vi "PCO_Convert.vi"() -> (1 "Raw_Length":u16, 4 "Length":u16, 6 "PCO_ConvertRaw_x64":T2, 7 "PCO_ConvertRaw_win32":T1, 8 "PCO_Convert":T3)   [LabVIEW 2019, in "Convert.lvlib"]
doc: "Use this template to build a VI to use as a subVI."
uses:
  Convert.lvlib
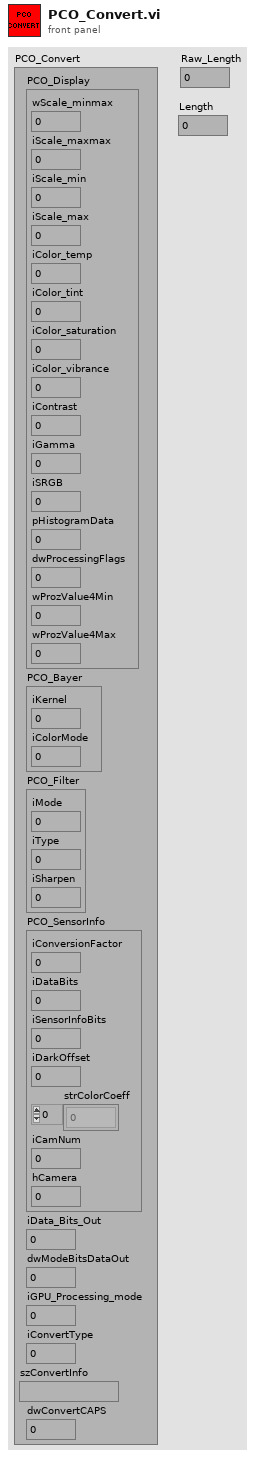
[diagram p1: front panel]
types:
  T1 = cluster{"wSize":u16, "wDummy":cluster{u16, u16, u16}, "PCO_DisplayRaw_win32":cluster{"wSize":u16, "wScale_minmax":u16, "iScale_maxmax":i32, "iScale_min":i32, "iScale_max":i32, "iColor_temp":i32, "iColor_tint":i32, "iColor_saturation":i32, "iColor_vibrance":i32, "iContrast":i32, "iGamma":i32, "iSRGB":i32, "pHistogramData":u32, "dwDialogOpenFlags":u32, "dwProcessingFlags":u32, "wProzValue4Min":u16, "wProzValue4Max":u16, "dwzzDummy1":cluster{u32, u32, u32, u32, u32, u32, u32, u32, u32, u32, u32, u32, u32, u32, u32, u32, u32, u32, u32, u32, u32, u32, u32, u32, u32, u32, u32, u32, u32, u32, u32, u32, u32, u32, u32, u32, u32, u32, u32, u32, u32, u32, u32, u32, u32, u32, u32, u32, u32}}, "PCO_Bayer_Raw":cluster{"wSize":u16, "wDummy":u16, "iKernel":i32, "iColorMode":i32, "dwzzDummy1":cluster{u32, u32, u32, u32, u32, u32, u32, u32, u32, u32, u32, u32, u32, u32, u32, u32, u32, u32, u32, u32, u32, u32, u32, u32, u32, u32, u32, u32, u32, u32, u32, u32, u32, u32, u32, u32, u32, u32, u32, u32, u32, u32, u32, u32, u32, u32, u32, u32, u32, u32, u32, u32, u32, u32, u32, u32, u32, u32, u32, u32, u32}}, "PCO_Filter_Raw":cluster{"wSize":u16, "wDummy":u16, "iMode":i32, "iType":i32, "iSharpen":i32, "dwzzDummy1":cluster{u32, u32, u32, u32, u32, u32, u32, u32, u32, u32, u32, u32, u32, u32, u32, u32, u32, u32, u32, u32, u32, u32, u32, u32, u32, u32, u32, u32, u32, u32, u32, u32, u32, u32, u32, u32, u32, u32, u32, u32, u32, u32, u32, u32, u32, u32, u32, u32, u32, u32, u32, u32, u32, u32, u32, u32, u32, u32, u32, u32}}, "PCO_SensorInfo_Raw_win32":cluster{"wSize":u16, "wDummy":u16, "iConversionFactor":i32, "iDataBits":i32, "iSensorInfoBits":i32, "iDarkOffset":i32, "dwzzDummy0":u32, "strColorCoeff":cluster{dbl, dbl, dbl, dbl, dbl, dbl, dbl, dbl, dbl}, "iCamNum":i32, "hCamera":u32, "dwzzDummy1":cluster{u32, u32, u32, u32, u32, u32, u32, u32, u32, u32, u32, u32, u32, u32, u32, u32, u32, u32, u32, u32, u32, u32, u32, u32, u32, u32, u32, u32, u32, u32, u32, u32, u32, u32, u32, u32, u32, u32}}, "iData_Bits_Out":i32, "dwModeBitsDataOut":u32, "iGPU_Processing_mode":i32, "iConvertType":i32, "szConvertInfo":cluster{u8, u8, u8, u8, u8, u8, u8, u8, u8, u8, u8, u8, u8, u8, u8, u8, u8, u8, u8, u8, u8, u8, u8, u8, u8, u8, u8, u8, u8, u8, u8, u8, u8, u8, u8, u8, u8, u8, u8, u8, u8, u8, u8, u8, u8, u8, u8, u8, u8, u8, u8, u8, u8, u8, u8, u8, u8, u8, u8, u8}, "dwConvertCAPS":u32, "dwzzDummy1":cluster{u32, u32, u32, u32, u32, u32, u32, u32, u32, u32, u32, u32, u32, u32, u32, u32, u32, u32, u32, u32, u32, u32, u32, u32, u32, u32, u32, u32, u32, u32, u32, u32, u32, u32, u32, u32, u32, u32, u32, u32, u32, u32}}
  T2 = cluster{"wSize":u16, "wDummy":cluster{u16, u16, u16}, "PCO_DisplayRaw_x64":cluster{"wSize":u16, "wScale_minmax":u16, "iScale_maxmax":i32, "iScale_min":i32, "iScale_max":i32, "iColor_temp":i32, "iColor_tint":i32, "iColor_saturation":i32, "iColor_vibrance":i32, "iContrast":i32, "iGamma":i32, "iSRGB":i32, "pHistogramData":u64, "dwDialogOpenFlags":u32, "dwProcessingFlags":u32, "wProzValue4Min":u16, "wProzValue4Max":u16, "dwzzDummy1":cluster{u32, u32, u32, u32, u32, u32, u32, u32, u32, u32, u32, u32, u32, u32, u32, u32, u32, u32, u32, u32, u32, u32, u32, u32, u32, u32, u32, u32, u32, u32, u32, u32, u32, u32, u32, u32, u32, u32, u32, u32, u32, u32, u32, u32, u32, u32, u32, u32, u32, u32}}, "PCO_Bayer_Raw":cluster{"wSize":u16, "wDummy":u16, "iKernel":i32, "iColorMode":i32, "dwzzDummy1":cluster{u32, u32, u32, u32, u32, u32, u32, u32, u32, u32, u32, u32, u32, u32, u32, u32, u32, u32, u32, u32, u32, u32, u32, u32, u32, u32, u32, u32, u32, u32, u32, u32, u32, u32, u32, u32, u32, u32, u32, u32, u32, u32, u32, u32, u32, u32, u32, u32, u32, u32, u32, u32, u32, u32, u32, u32, u32, u32, u32, u32, u32}}, "PCO_Filter_Raw":cluster{"wSize":u16, "wDummy":u16, "iMode":i32, "iType":i32, "iSharpen":i32, "dwzzDummy1":cluster{u32, u32, u32, u32, u32, u32, u32, u32, u32, u32, u32, u32, u32, u32, u32, u32, u32, u32, u32, u32, u32, u32, u32, u32, u32, u32, u32, u32, u32, u32, u32, u32, u32, u32, u32, u32, u32, u32, u32, u32, u32, u32, u32, u32, u32, u32, u32, u32, u32, u32, u32, u32, u32, u32, u32, u32, u32, u32, u32, u32}}, "PCO_SensorInfo_Raw_x64":cluster{"wSize":u16, "wDummy":u16, "iConversionFactor":i32, "iDataBits":i32, "iSensorInfoBits":i32, "iDarkOffset":i32, "dwzzDummy0":u32, "strColorCoeff":cluster{dbl, dbl, dbl, dbl, dbl, dbl, dbl, dbl, dbl}, "iCamNum":i32, "hCamera":u64, "dwzzDummy1":cluster{u32, u32, u32, u32, u32, u32, u32, u32, u32, u32, u32, u32, u32, u32, u32, u32, u32, u32, u32, u32, u32, u32, u32, u32, u32, u32, u32, u32, u32, u32, u32, u32, u32, u32, u32, u32, u32, u32, u32}}, "iData_Bits_Out":i32, "dwModeBitsDataOut":u32, "iGPU_Processing_mode":i32, "iConvertType":i32, "szConvertInfo":cluster{u8, u8, u8, u8, u8, u8, u8, u8, u8, u8, u8, u8, u8, u8, u8, u8, u8, u8, u8, u8, u8, u8, u8, u8, u8, u8, u8, u8, u8, u8, u8, u8, u8, u8, u8, u8, u8, u8, u8, u8, u8, u8, u8, u8, u8, u8, u8, u8, u8, u8, u8, u8, u8, u8, u8, u8, u8, u8, u8, u8}, "dwConvertCAPS":u32, "dwzzDummy1":cluster{u32, u32, u32, u32, u32, u32, u32, u32, u32, u32, u32, u32, u32, u32, u32, u32, u32, u32, u32, u32, u32, u32, u32, u32, u32, u32, u32, u32, u32, u32, u32, u32, u32, u32, u32, u32, u32, u32, u32, u32, u32, u32}}
  T3 = cluster{"PCO_Display":cluster{"wScale_minmax":u16, "iScale_maxmax":i32, "iScale_min":i32, "iScale_max":i32, "iColor_temp":i32, "iColor_tint":i32, "iColor_saturation":i32, "iColor_vibrance":i32, "iContrast":i32, "iGamma":i32, "iSRGB":i32, "pHistogramData":u64, "dwProcessingFlags":u32, "wProzValue4Min":u16, "wProzValue4Max":u16}, "PCO_Bayer":cluster{"iKernel":i32, "iColorMode":i32}, "PCO_Filter":cluster{"iMode":i32, "iType":i32, "iSharpen":i32}, "PCO_SensorInfo":cluster{"iConversionFactor":i32, "iDataBits":i32, "iSensorInfoBits":i32, "iDarkOffset":i32, "strColorCoeff":dbl[], "iCamNum":i32, "hCamera":u64}, "iData_Bits_Out":i32, "dwModeBitsDataOut":u32, "iGPU_Processing_mode":i32, "iConvertType":i32, "szConvertInfo":string, "dwConvertCAPS":u32}
  T4 = cluster{u8, u8, u8, u8, u8, u8, u8, u8, u8, u8, u8, u8, u8, u8, u8, u8, u8, u8, u8, u8, u8, u8, u8, u8, u8, u8, u8, u8, u8, u8, u8, u8, u8, u8, u8, u8, u8, u8, u8, u8, u8, u8, u8, u8, u8, u8, u8, u8, u8, u8, u8, u8, u8, u8, u8, u8, u8, u8, u8, u8}
  T5 = cluster{u32, u32, u32, u32, u32, u32, u32, u32, u32, u32, u32, u32, u32, u32, u32, u32, u32, u32, u32, u32, u32, u32, u32, u32, u32, u32, u32, u32, u32, u32, u32, u32, u32, u32, u32, u32, u32, u32, u32, u32, u32, u32}
  T6 = cluster{"wSize":u16, "wScale_minmax":u16, "iScale_maxmax":i32, "iScale_min":i32, "iScale_max":i32, "iColor_temp":i32, "iColor_tint":i32, "iColor_saturation":i32, "iColor_vibrance":i32, "iContrast":i32, "iGamma":i32, "iSRGB":i32, "pHistogramData":u64, "dwDialogOpenFlags":u32, "dwProcessingFlags":u32, "wProzValue4Min":u16, "wProzValue4Max":u16, "dwzzDummy1":cluster{u32, u32, u32, u32, u32, u32, u32, u32, u32, u32, u32, u32, u32, u32, u32, u32, u32, u32, u32, u32, u32, u32, u32, u32, u32, u32, u32, u32, u32, u32, u32, u32, u32, u32, u32, u32, u32, u32, u32, u32, u32, u32, u32, u32, u32, u32, u32, u32, u32, u32}}
  T7 = cluster{"wScale_minmax":u16, "iScale_maxmax":i32, "iScale_min":i32, "iScale_max":i32, "iColor_temp":i32, "iColor_tint":i32, "iColor_saturation":i32, "iColor_vibrance":i32, "iContrast":i32, "iGamma":i32, "iSRGB":i32, "pHistogramData":u64, "dwProcessingFlags":u32, "wProzValue4Min":u16, "wProzValue4Max":u16}
  T8 = cluster{"wSize":u16, "wScale_minmax":u16, "iScale_maxmax":i32, "iScale_min":i32, "iScale_max":i32, "iColor_temp":i32, "iColor_tint":i32, "iColor_saturation":i32, "iColor_vibrance":i32, "iContrast":i32, "iGamma":i32, "iSRGB":i32, "pHistogramData":u32, "dwDialogOpenFlags":u32, "dwProcessingFlags":u32, "wProzValue4Min":u16, "wProzValue4Max":u16, "dwzzDummy1":cluster{u32, u32, u32, u32, u32, u32, u32, u32, u32, u32, u32, u32, u32, u32, u32, u32, u32, u32, u32, u32, u32, u32, u32, u32, u32, u32, u32, u32, u32, u32, u32, u32, u32, u32, u32, u32, u32, u32, u32, u32, u32, u32, u32, u32, u32, u32, u32, u32, u32}}
  T9 = cluster{"wSize":u16, "wDummy":u16, "iKernel":i32, "iColorMode":i32, "dwzzDummy1":cluster{u32, u32, u32, u32, u32, u32, u32, u32, u32, u32, u32, u32, u32, u32, u32, u32, u32, u32, u32, u32, u32, u32, u32, u32, u32, u32, u32, u32, u32, u32, u32, u32, u32, u32, u32, u32, u32, u32, u32, u32, u32, u32, u32, u32, u32, u32, u32, u32, u32, u32, u32, u32, u32, u32, u32, u32, u32, u32, u32, u32, u32}}
  T10 = cluster{"iMode":i32, "iType":i32, "iSharpen":i32}
  T11 = cluster{"wSize":u16, "wDummy":u16, "iMode":i32, "iType":i32, "iSharpen":i32, "dwzzDummy1":cluster{u32, u32, u32, u32, u32, u32, u32, u32, u32, u32, u32, u32, u32, u32, u32, u32, u32, u32, u32, u32, u32, u32, u32, u32, u32, u32, u32, u32, u32, u32, u32, u32, u32, u32, u32, u32, u32, u32, u32, u32, u32, u32, u32, u32, u32, u32, u32, u32, u32, u32, u32, u32, u32, u32, u32, u32, u32, u32, u32, u32}}
  T12 = cluster{"wSize":u16, "wDummy":u16, "iConversionFactor":i32, "iDataBits":i32, "iSensorInfoBits":i32, "iDarkOffset":i32, "dwzzDummy0":u32, "strColorCoeff":cluster{dbl, dbl, dbl, dbl, dbl, dbl, dbl, dbl, dbl}, "iCamNum":i32, "hCamera":u64, "dwzzDummy1":cluster{u32, u32, u32, u32, u32, u32, u32, u32, u32, u32, u32, u32, u32, u32, u32, u32, u32, u32, u32, u32, u32, u32, u32, u32, u32, u32, u32, u32, u32, u32, u32, u32, u32, u32, u32, u32, u32, u32, u32}}
  T13 = cluster{"iConversionFactor":i32, "iDataBits":i32, "iSensorInfoBits":i32, "iDarkOffset":i32, "strColorCoeff":dbl[], "iCamNum":i32, "hCamera":u64}
  T14 = cluster{"wSize":u16, "wDummy":u16, "iConversionFactor":i32, "iDataBits":i32, "iSensorInfoBits":i32, "iDarkOffset":i32, "dwzzDummy0":u32, "strColorCoeff":cluster{dbl, dbl, dbl, dbl, dbl, dbl, dbl, dbl, dbl}, "iCamNum":i32, "hCamera":u32, "dwzzDummy1":cluster{u32, u32, u32, u32, u32, u32, u32, u32, u32, u32, u32, u32, u32, u32, u32, u32, u32, u32, u32, u32, u32, u32, u32, u32, u32, u32, u32, u32, u32, u32, u32, u32, u32, u32, u32, u32, u32, u32}}
  T15 = cluster{"PCO_Display":cluster{"wScale_minmax":u16, "iScale_maxmax":i32, "iScale_min":i32, "iScale_max":i32, "iColor_temp":i32, "iColor_tint":i32, "iColor_saturation":i32, "iColor_vibrance":i32, "iContrast":i32, "iGamma":i32, "iSRGB":i32, "pHistogramData":u64, "dwProcessingFlags":u32, "wProzValue4Min":u16, "wProzValue4Max":u16}, "PCO_Bayer":cluster{"iKernel":i32, "iColorMode":i32}, "PCO_Filter":cluster{"iMode":i32, "iType":i32, "iSharpen":i32}, "PCO_SensorInfo":cluster{"iConversionFactor":i32, "iDataBits":i32, "iSensorInfoBits":i32, "iDarkOffset":i32, "strColorCoeff":dbl[], "iCamNum":i32, "hCamera":u64}, "iData_Bits_Out":i32, "dwModeBitsDataOut":u32, "iGPU_Processing_mode":i32, "iConvertType":i32, "string":string, "dwConvertCAPS":u32}
  T16 = enum8{"Enabled", "Disabled", "Disabled and Grayed Out"}
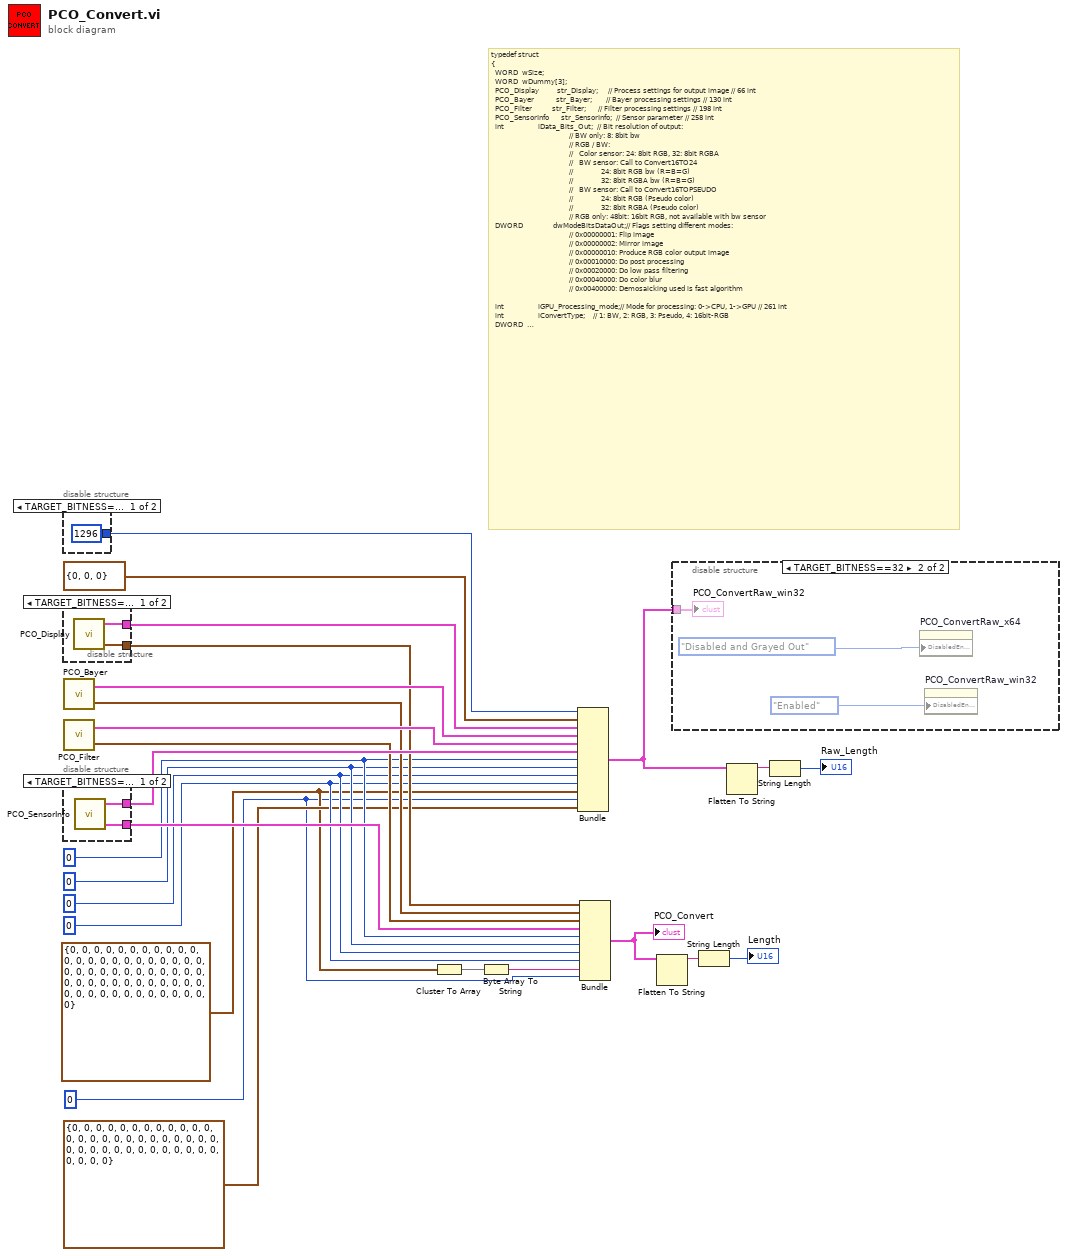
[diagram p0: block diagram]
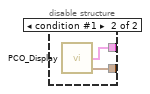
[diagram p2: hidden frame]
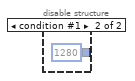
[diagram p3: hidden frame]
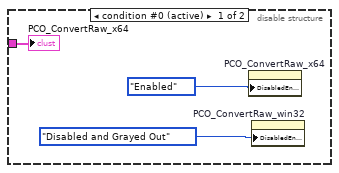
[diagram p4: hidden frame]
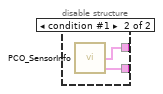
[diagram p5: hidden frame]
diagram:
  w3 = T4 {0, 0, 0, 0, 0, 0, 0, 0, 0, 0, 0, 0, 0, 0, 0, 0, 0, 0, 0, 0, 0, 0, 0, 0, 0, 0, 0, 0, 0, 0, 0, 0, 0, 0, 0, 0, 0, 0, 0, 0, 0, 0, 0, 0, 0, 0, 0, 0, 0, 0, 0, 0, 0, 0, 0, 0, 0, 0, 0, 0} ("szConvertInfo")
  w1 = u32 0 ("dwConvertCAPS")
  w9 = 0 ("iData_Bits_Out")
  w8 = u32 0 ("dwModeBitsDataOut")
  w7 = 0 ("iGPU_Processing_mode")
  w6 = 0 ("iConvertType")
  # "typedef struct \n{\n  WORD  wSize;\n  WORD  wDummy[3];\n  PCO_Display         str_Display;     // Process settings for output image // 66 int\n  PCO_Bayer           str_Bayer;       // Bayer processing settings // 130 int\n  PCO_Filter          str_Filter;      // Filter processing settings // 198 int\n  PCO_SensorInfo      str_SensorInfo;  // Sensor parameter // 258 int\n  int                 iData_Bits_Out;  // Bit resolution of output:\n                                       // BW only: 8: 8bit bw\n                                       // RGB / BW:\n                                       //   Color sensor: 24: 8bit RGB, 32: 8bit RGBA\n                                       //   BW sensor: Call to Convert16TO24\n                                       //              24: 8bit RGB bw (R=B=G)\n                                       //              32: 8bit RGBA bw (R=B=G)\n                                       //   BW sensor: Call to Convert16TOPSEUDO\n                                       //              24: 8bit RGB (Pseudo color)\n                                       //              32: 8bit RGBA (Pseudo color)\n                                       // RGB only: 48bit: 16bit RGB, not available with bw sensor\n  DWORD               dwModeBitsDataOut;// Flags setting different modes:\n                                       // 0x00000001: Flip image\n                                       // 0x00000002: Mirror image\n                                       // 0x00000010: Produce RGB color output image\n                                       // 0x00010000: Do post processing\n                                       // 0x00020000: Do low pass filtering\n                                       // 0x00040000: Do color blur\n                                       // 0x00400000: Demosaicking used is fast algorithm\n\n  int                 iGPU_Processing_mode;// Mode for processing: 0->CPU, 1->GPU // 261 int\n  int                 iConvertType;    // 1: BW, 2: RGB, 3: Pseudo, 4: 16bit-RGB\n  DWORD               dwzzDummy1[58];  // 320 int\n}PCO_Convert;"
  n1 = disable-structure "Diagram Disable Structure" shown="TARGET_BITNESS==64, Default" {
    disable-tunnel: [u16 1296 ("wSize") u16 1280 ("wSize")] -> w19
    frame condition #0 (active) {
    }
    frame condition #1 {
    }
  }
  n2 = disable-structure "Diagram Disable Structure" shown="TARGET_BITNESS==64, Standard" {
    disable-tunnel: [w29 w31] -> w17
    disable-tunnel: [w28 w30] -> w13
    frame condition #0 (active) {
      n3 = call "PCO_Display.vi"() -> ("PCO_DisplayRaw_x64"=w29:T6, "PCO_Display"=w28:T7)  [unwired: 4 in, 3 out]
    }
    frame condition #1 {
      n4 = call "PCO_Display.vi"() -> ("PCO_DisplayRaw_win32"=w31:T8, "PCO_Display"=w30:T7)  [unwired: 4 in, 3 out]
    }
  }
  n5 = call "PCO_Bayer.vi"() -> ("PCO_Bayer"=w12:cluster{"iKernel":i32, "iColorMode":i32}, "PCO_Bayer_Raw"=w16:T9)  [unwired: 4 in, 2 out]
  n6 = call "PCO_Filter.vi"() -> ("PCO_Filter"=w11:T10, "PCO_Filter_Raw"=w15:T11)  [unwired: 4 in, 2 out]
  n7 = disable-structure "Diagram Disable Structure" shown="TARGET_BITNESS==64, Standard" {
    disable-tunnel: [w33 w35] -> w14
    disable-tunnel: [w32 w34] -> w10
    frame condition #0 (active) {
      n8 = call "PCO_SensorInfo.vi"() -> ("PCO_SensorInfo_Raw_x64"=w33:T12, "PCO_SensorInfo"=w32:T13)  [unwired: 4 in, 3 out]
    }
    frame condition #1 {
      n9 = call "PCO_SensorInfo.vi"() -> ("PCO_SensorInfo_Raw_win32"=w35:T14, "PCO_SensorInfo"=w34:T13)  [unwired: 4 in, 3 out]
    }
  }
  n10 = Cluster To Array(cluster=w3) -> (array=w2:u8[])
  n11 = Byte Array To String(unsigned byte array=w2) -> (string=w4:string)
  n12 = Bundle("wSize"=w19, "wDummy"=cluster{u16, u16, u16} {0, 0, 0}, "PCO_DisplayRaw_x64"=w17, "PCO_Bayer_Raw"=w16, "PCO_Filter_Raw"=w15, "PCO_SensorInfo_Raw_x64"=w14, "iData_Bits_Out"=w9, "dwModeBitsDataOut"=w8, "iGPU_Processing_mode"=w7, "iConvertType"=w6, "szConvertInfo"=w3, "dwConvertCAPS"=w1, "dwzzDummy1"=T5 {0, 0, 0, 0, 0, 0, 0, 0, 0, 0, 0, 0, 0, 0, 0, 0, 0, 0, 0, 0, 0, 0, 0, 0, 0, 0, 0, 0, 0, 0, 0, 0, 0, 0, 0, 0, 0, 0, 0, 0, 0, 0}) -> (w20:T2)  [unwired: 1 in]
  n13 = Bundle("PCO_Display"=w13, "PCO_Bayer"=w12, "PCO_Filter"=w11, "PCO_SensorInfo"=w10, "iData_Bits_Out"=w9, "dwModeBitsDataOut"=w8, "iGPU_Processing_mode"=w7, "iConvertType"=w6, "string"=w4, "dwConvertCAPS"=w1) -> (w25:T15)  [unwired: 1 in]
  "PCO_Convert" <- w25
  n14 = Flatten To String(anything=w25) -> (data string=w24:string)  [unwired: 3 in, 2 out]
  n15 = disable-structure "Diagram Disable Structure" shown="TARGET_BITNESS==32" {
    disable-tunnel: w20 -> [w38 w40]
    frame condition #0 (active) {
      n16 = property on="PCO_ConvertRaw_x64" class="Clust (strict)"("DisabledEnum"=T16."Enabled" ("Disabled")) -> ()  [unwired: 2 in, 2 out]
      n17 = property on="PCO_ConvertRaw_win32" class="Clust (strict)"("DisabledEnum"=T16."Disabled and Grayed Out" ("Disabled")) -> ()  [unwired: 2 in, 2 out]
      "PCO_ConvertRaw_x64" <- w38
    }
    frame condition #1 {
      n18 = property on="PCO_ConvertRaw_x64" class="Clust (strict)"("DisabledEnum"=T16."Disabled and Grayed Out" ("Disabled")) -> ()  [unwired: 2 in, 2 out]
      n19 = property on="PCO_ConvertRaw_win32" class="Clust (strict)"("DisabledEnum"=T16."Enabled" ("Disabled")) -> ()  [unwired: 2 in, 2 out]
      "PCO_ConvertRaw_win32" <- w40
    }
  }
  n20 = String Length(string=w24) -> (length=→"Length":i32)
  n21 = Flatten To String(anything=w20) -> (data string=w23:string)  [unwired: 3 in, 2 out]
  n22 = String Length(string=w23) -> (length=→"Raw_Length":i32)
